vi "FCI_Lip_Gap_Plus_Lip_Level_Pats.vi"(0 "Image":T7(plugin-control), 1 "Calibrated Image":T7, 2 "Ref ROI":T2 {"Contours"."Type" items=["No Selection", "Point", "Line", "Rectangle", "Oval", "Polygon", "Freehand Region", "Annulus", "Unused2", "Unused3", "Broken Line", "Freehand Line", "Rotated Rectangle"]}, 3 "Measurement ROI 1":T2 {"Contours"."Type" items=["No Selection", "Point", "Line", "Rectangle", "Oval", "Polygon", "Freehand Region", "Annulus", "Unused2", "Unused3", "Broken Line", "Freehand Line", "Rotated Rectangle"]}, 4 "Measurement ROI 2":T2 {"Contours"."Type" items=["No Selection", "Point", "Line", "Rectangle", "Oval", "Polygon", "Freehand Region", "Annulus", "Unused2", "Unused3", "Broken Line", "Freehand Line", "Rotated Rectangle"]}, 5 "Line Options Ref ROI":T5={"Number of Lines"=1, "Type"=enum."First Edge Rake", "Min. Score"=10.0, "Max. Score"=1000.0, "Orientation"=0.0, "Angle Range"=45.0, "Angle Tolerance"=1.0, "Step Size"=5, "Min. SNR (db)"=0.0, "Min. Points (%)"=25.0, "Hough Iterations"=5} {"Min. Points (%)" min=0.0 max=100.0; "Min. SNR (db)" min=0.0; "Max. Score" min=0.0 max=1024.0; "Min. Score" min=0.0 max=1024.0 step=1.0}, 6 "Search Direction Ref ROI":u32=2, 7 "error in (no error)":errorcluster, 8 "Search Direction ROI 1":u16(ring) items=["Left To Right", "Right To Left", "Top To Bottom", "Bottom To Top"], 9 "Edge Options ROI 1":T3={"Edge Polarity"=0, "Kernel Size"=3, "Width"=3, "Minimum Edge Strength"=50.0, "Interpolation Type"=enum."Zero Order", "Data Processing Method"=enum."Average"} {"Edge Polarity" items=["All Edges", "Rising Edges", "Falling Edges"]; "Minimum Edge Strength" format="%.2f"; "Width" step=2; "Kernel Size" step=2}, 10 "Search Direction ROI 2":u16(ring)=2 items=["Left To Right", "Right To Left", "Top To Bottom", "Bottom To Top"], 11 "Process ROI 2":T1(ring), 12 "Step Size ROI 2":u32=2, 13 "Edge Options Ref ROI":T3={"Edge Polarity"=0, "Kernel Size"=3, "Width"=3, "Minimum Edge Strength"=40.0, "Interpolation Type"=enum."Zero Order", "Data Processing Method"=enum."Average"} {"Edge Polarity" items=["All Edges", "Rising Edges", "Falling Edges"]; "Minimum Edge Strength" format="%.2f"; "Width" step=2; "Kernel Size" step=2}) -> (20 "Real World Lip Level":sgl, 27 "error IO":errorcluster)   [LabVIEW 2019, in "Algorithm.lvclass"]
uses:
  FrameworkOverrides/Algorithm.lvclass
  <vilib>/vision/NI_Vision_Development_Module.lvlib
  <vilib>/vision/Measure.llb/Edge Polarity.ctl
  <vilib>/vision/Measure.llb/Edge Options.ctl
  <vilib>/vision/Image Controls.llb/IMAQ Image.ctl
  <vilib>/vision/Measure.llb/Straight Edge Process.ctl
  <vilib>/vision/Measure.llb/Straight Edge Options.ctl
panel:
  out "Y1":sgl
  out "Y2":sgl
  out "Pixel Level Difference":sgl
  out "Point 2":cluster{"X":sgl, "Y":sgl}
  out "Point 1":cluster{"X":sgl, "Y":sgl}
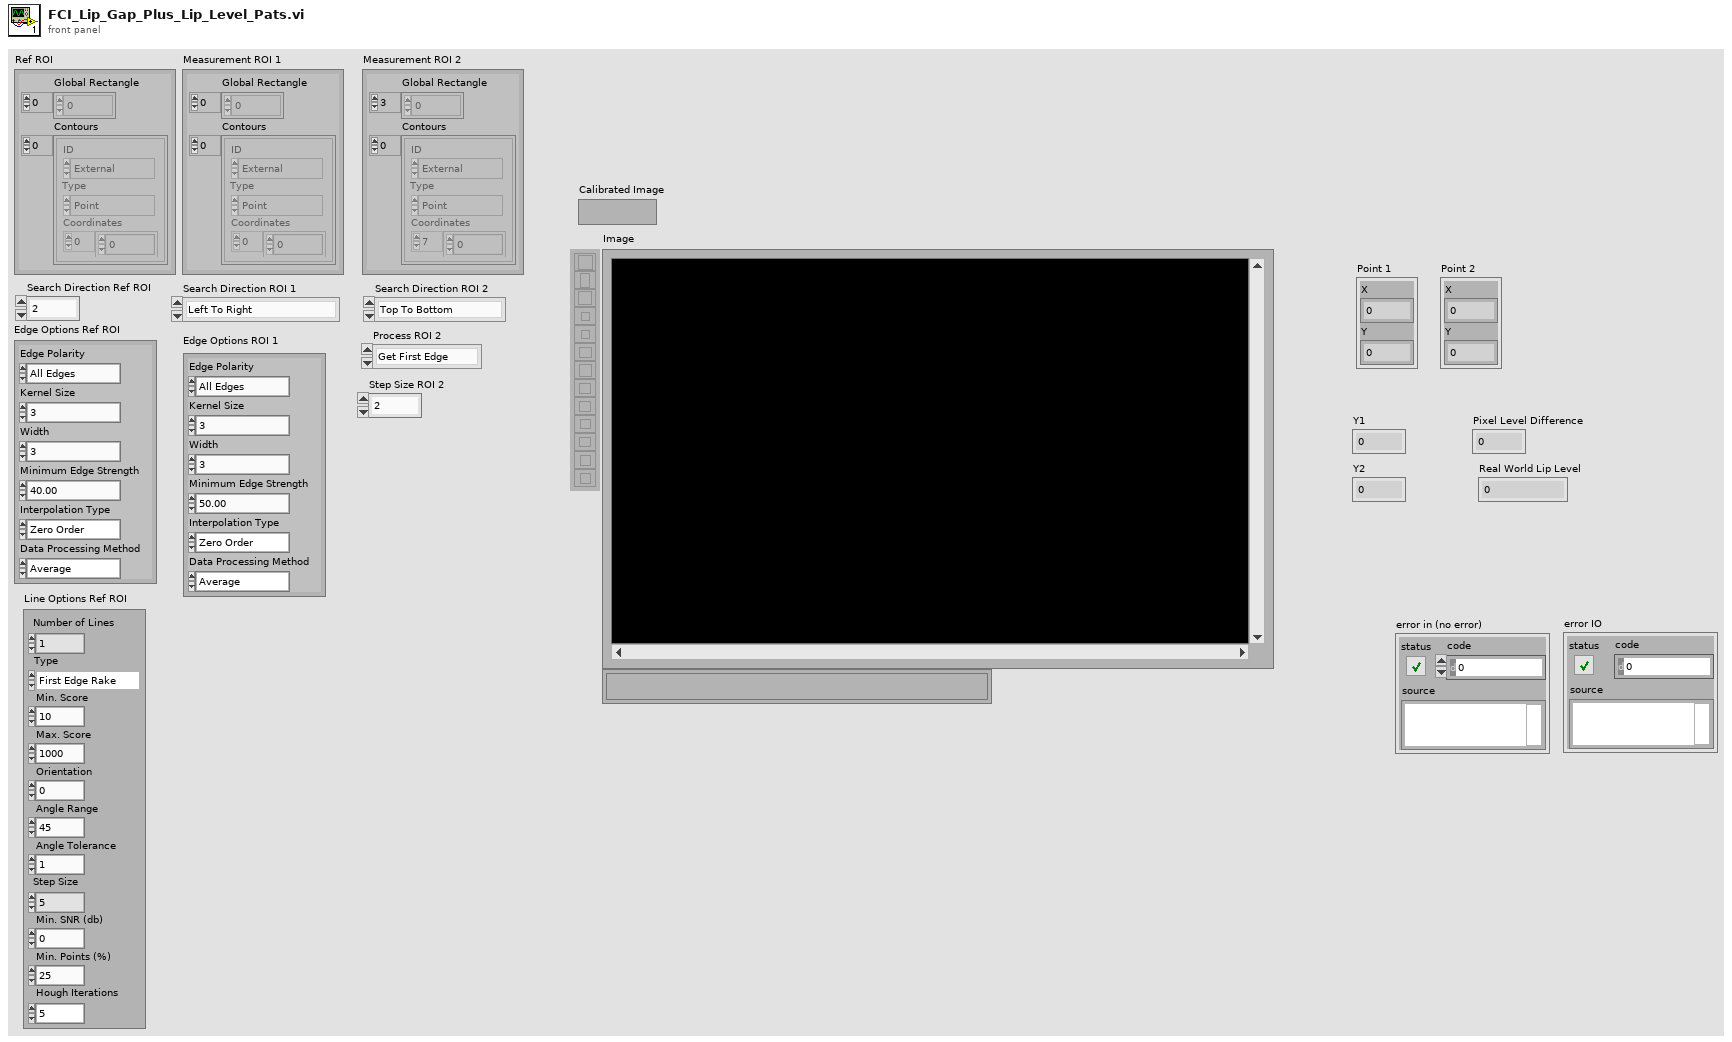
[diagram p1: front panel]
types:
  T1 = enum16{"Get First Edge", "Get First + Last Edge", "Get All Edges", "Get Best Edge"}
  T2 = typedef "ROI Descriptor" = cluster{"Global Rectangle":i32[], "Contours":cluster{"ID":enum32{"External", "Internal"}, "Type":u32, "Coordinates":i32[]}[]}
  T3 = typedef "Edge Options.ctl" = cluster{"Edge Polarity":T4, "Kernel Size":u32, "Width":u32, "Minimum Edge Strength":sgl, "Interpolation Type":enum32{"Zero Order", "Bilinear", "Quadratic", "Cubic", "Bilinear Fixed"}, "Data Processing Method":enum32{"Average", "Median"}}
  T4 = typedef "Edge Polarity.ctl" = u32
  T5 = typedef "Straight Edge Options.ctl" = cluster{"Number of Lines":i32, "Type":T6, "Min. Score":dbl, "Max. Score":dbl, "Orientation":dbl, "Angle Range":dbl, "Angle Tolerance":dbl, "Step Size":u32, "Min. SNR (db)":dbl, "Min. Points (%)":dbl, "Hough Iterations":i32}
  T6 = typedef "Straight Edge Process.ctl" = enum32{"First Edge Rake", "Best Edge Rake", "Hough Edge Rake", "First Edge Projection", "Best Edge Projection"}
  T7 = typedef "IMAQ Image.ctl" = refnum<image>
  T8 = cluster{"Left":dbl, "Top":dbl, "Right":dbl, "Bottom":dbl, "Angle":dbl}
  T9 = cluster{"Search Direction":u32, "Edge Options":T3, "Show Search Area":bool, "Show Search Lines":bool, "Show Edges Found":bool, "Show Result":bool, "Search Area Color":u32, "Search Lines Color":u32, "Edge Locations Color":u32, "Result Color":u32, "Overlay Group Name":string}
  T10 = typedef "IMAQ Rectangle" = cluster{"Left":i32, "Top":i32, "Right":i32, "Bottom":i32, "Rotation":dbl}
  T11 = cluster{"Point1 (Pixels)":cluster{"X":sgl, "Y":sgl}, "Point2 (Pixels)":cluster{"X":sgl, "Y":sgl}, "Point1 (Real-World)":cluster{"X":sgl, "Y":sgl}, "Point2 (Real-World)":cluster{"X":sgl, "Y":sgl}, "Angle (Pixel)":dbl, "Angle (Real-World)":dbl, "Score":dbl, "Straightness":dbl, "Average SNR (db)":dbl, "Calibration Valid":bool}[]
  T12 = cluster{"Point1 (Pixels)":cluster{"X":sgl, "Y":sgl}, "Point2 (Pixels)":cluster{"X":sgl, "Y":sgl}, "Point1 (Real-World)":cluster{"X":sgl, "Y":sgl}, "Point2 (Real-World)":cluster{"X":sgl, "Y":sgl}, "Angle (Pixel)":dbl, "Angle (Real-World)":dbl, "Score":dbl, "Straightness":dbl, "Average SNR (db)":dbl, "Calibration Valid":bool}
  T13 = typedef "Edge New.ctl" = cluster{"Location (Pixel)":cluster{"X":sgl, "Y":sgl}, "Location (Real-World)":cluster{"X":sgl, "Y":sgl}, "Distance (Pixel)":dbl, "Distance (Real-World)":dbl, "Strength":dbl, "Noise":dbl, "Rising?":bool}
  T14 = cluster{cluster{"X":sgl, "Y":sgl}, cluster{"X":sgl, "Y":sgl}}
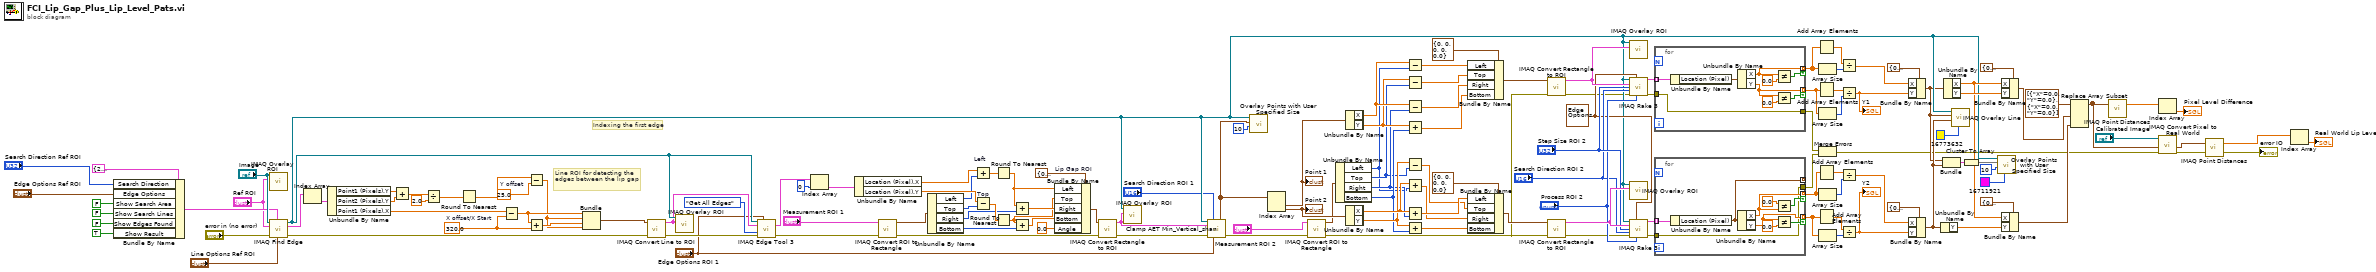
[diagram p0: block diagram]
diagram:
  w56 = sgl 25.0  # Y offset
  w64 = sgl 320.0  # X offset/X Start
  w129 = T3 {"Edge Polarity"=2, "Kernel Size"=3, "Width"=3, "Minimum Edge Strength"=50.0, "Interpolation Type"=enum."Zero Order", "Data Processing Method"=enum."Average"} ("Edge Options")
  # "Indexing the first edge"
  # "Line ROI for detecting the edges between the lip gap"
  n1 = Bundle By Name(cluster=T9 {"Search Direction"=2, "Edge Options"={"Edge Polarity"=0, "Kernel Size"=3, "Width"=3, "Minimum Edge Strength"=40.0, "Interpolation Type"=enum."Zero Order", "Data Processing Method"=enum."Average"}, "Show Search Area"=FALSE, "Show Search Lines"=FALSE, "Show Edges Found"=FALSE, "Show Result"=TRUE, "Search Area Color"=65280, "Search Lines Color"=255, "Edge Locations Color"=16776960, "Result Color"=16711680, "Overlay Group Name"=""} ("Options"), "Search Direction"="Search Direction Ref ROI", "Edge Options"="Edge Options Ref ROI", "Show Search Area"=FALSE, "Show Search Lines"=FALSE, "Show Edges Found"=FALSE, "Show Result"=TRUE) -> (w34:T9)
  n2 = call "IMAQ Overlay ROI"("ROI Descriptor"="Ref ROI", "Image"="Image") -> ()  [unwired: 8 in, 2 out]
  n3 = call "IMAQ Find Edge"("Line Fit Options"="Line Options Ref ROI", "Options"=w34, "error in (no error)"="error in (no error)", "ROI Descriptor"="Ref ROI", "Image"="Image") -> ("error out"=w62:errorcluster, "Straight Edges"=w74:T11, "Image Out"=w80:T7)  [unwired: 3 in, 1 out]
  n4 = Index Array(array=w74) -> (element=w73:T12)  [unwired: 1 in]
  n5 = Unbundle By Name(w73) -> ("Point1 (Pixels).Y"=w72:sgl, "Point2 (Pixels).Y"=w71:sgl, "Point1 (Pixels).X"=w67:sgl)
  n6 = Add(x=w72, y=w71) -> (x+y=w70:sgl)
  n7 = Divide(x=w70, y=sgl 2.0) -> (x/y=w68:sgl)
  n8 = Round To Nearest(number=w68) -> (nearest integer value=w57:sgl)
  n9 = Subtract(x=w67, y=w64) -> (x-y=w66:sgl)
  n10 = Subtract(x=w57, y=w56) -> (x-y=w58:sgl)
  n11 = Add(x=w66, y=w64) -> (x+y=w65:sgl)
  n12 = Bundle(w66, w58, w65, w58) -> (w63:cluster{sgl, sgl, sgl, sgl})  [unwired: 1 in]
  n13 = call "IMAQ Convert Line to ROI"("error in (no error)"=w62, "Line"=w63) -> ("error out"=w61:errorcluster, "ROI Descriptor"=w59:T2)  [unwired: 7 in]
  n14 = call "IMAQ Overlay ROI"("ROI Descriptor"=w59, "Image"=w80) -> ()  [unwired: 8 in, 2 out]
  n15 = call "IMAQ Edge Tool 3"("Image"=w80, "Edge Options"="Edge Options ROI 1", "ROI Descriptor"=w59, "Process"=T1."Get All Edges", "error in (no error)"=w61) -> ("Edge Information"=w55:T13[], "error out"=w21:errorcluster)  [unwired: 6 in, 3 out]
  n16 = Index Array(array=w55, index=0) -> (element=w54:T13)
  n17 = Unbundle By Name(w54) -> ("Location (Pixel).X"=w51:sgl, "Location (Pixel).Y"=w50:sgl)
  n18 = call "IMAQ Convert ROI to Rectangle"("error in (no error)"=w21, "ROI Descriptor"="Measurement ROI 1") -> ("error out"=w20:errorcluster, "Rectangle"=w27:T10)  [unwired: 7 in]
  n19 = Unbundle By Name(w27) -> ("Left"=w26:i32, "Top"=w25:i32, "Right"=w24:i32, "Bottom"=w23:i32)
  n20 = Add "Left"(x=w51, y=w26) -> (x+y=w49:sgl)
  n21 = Subtract "Top"(x=w50, y=w25) -> (x-y=w48:sgl)
  n22 = Round To Nearest(number=w49) -> (nearest integer value=w46:sgl)
  n23 = Round To Nearest(number=w48) -> (nearest integer value=w44:sgl)
  n24 = Add(x=w46, y=w24) -> (x+y=w45:sgl)
  n25 = Add(x=w44, y=w23) -> (x+y=w43:sgl)
  n26 = Bundle By Name "Lip Gap ROI"(cluster=T8 {"Left"=0.0, "Top"=0.0, "Right"=0.0, "Bottom"=0.0, "Angle"=0.0} ("input cluster"), "Left"=w46, "Top"=w44, "Right"=w45, "Bottom"=w43, "Angle"=0.0) -> (w47:T8)
  n27 = call "IMAQ Convert Rectangle to ROI"("error in (no error)"=w20, "Rectangle"=w47) -> ("error out"=w42:errorcluster, "ROI Descriptor"=w41:T2)  [unwired: 7 in]
  n28 = call "IMAQ Overlay ROI"("ROI Descriptor"=w41, "Image"=w80) -> ()  [unwired: 8 in, 2 out]
  n29 = call "Clamp AET Min_Vertical_shan.vi"("Image"=w80, "Scanning axis"="Search Direction ROI 1", "ROI Descriptor"=w41, "error in (no error)"=w42, "Edge Options"="Edge Options ROI 1") -> ("Edge Coordinates"=w141:cluster{"X":sgl, "Y":sgl}[], "error out"=w9:errorcluster)  [unwired: 4 in, 5 out]
  n30 = call "Overlay Points with User Specified Size.vi"("Point Diameter (5)"=u32 10, "Points"=w141, "Image In"=w80) -> ()  [unwired: 7 in, 2 out]
  n31 = Index Array(array=w141) -> (element #1=w140:cluster{"X":sgl, "Y":sgl}, element #2=w137:cluster{"X":sgl, "Y":sgl})  [unwired: 2 in]
  "Point 1" <- w140
  "Point 2" <- w137
  n32 = call "IMAQ Convert ROI to Rectangle"("error in (no error)"=w9, "ROI Descriptor"="Measurement ROI 2") -> ("error out"=w8:errorcluster, "Rectangle"=w7:T10)  [unwired: 7 in]
  n33 = Unbundle By Name(w7) -> ("Left"=w3:i32, "Top"=w4:i32, "Right"=w5:i32, "Bottom"=w6:i32)
  n34 = Unbundle By Name(w140) -> ("X"=w90:sgl, "Y"=w81:sgl)
  n35 = Unbundle By Name(w137) -> ("X"=w86:sgl, "Y"=w84:sgl)
  n36 = Subtract(x=w90, y=w3) -> (x-y=w91:sgl)
  n37 = Subtract(x=w81, y=w4) -> (x-y=w85:sgl)
  n38 = Subtract(x=w90, y=w5) -> (x-y=w89:sgl)
  n39 = Add(x=w81, y=w6) -> (x+y=w82:sgl)
  n40 = Subtract(x=w84, y=w4) -> (x-y=w83:sgl)
  n41 = Add(x=w86, y=w3) -> (x+y=w2:sgl)
  n42 = Add(x=w86, y=w5) -> (x+y=w88:sgl)
  n43 = Add(x=w84, y=w6) -> (x+y=w87:sgl)
  n44 = Bundle By Name(cluster=T10 {"Left"=0, "Top"=0, "Right"=0, "Bottom"=0, "Rotation"=0.0} ("Rectangle"), "Left"=w91, "Top"=w85, "Right"=w89, "Bottom"=w82) -> (w138:T10)
  n45 = Bundle By Name(cluster=T10 {"Left"=0, "Top"=0, "Right"=0, "Bottom"=0, "Rotation"=0.0} ("Rectangle"), "Left"=w88, "Top"=w83, "Right"=w2, "Bottom"=w87) -> (w135:T10)
  n46 = call "IMAQ Convert Rectangle to ROI"("error in (no error)"=w8, "Rectangle"=w138) -> ("error out"=w17:errorcluster, "ROI Descriptor"=w134:T2)  [unwired: 7 in]
  n47 = call "IMAQ Convert Rectangle to ROI"("error in (no error)"=w8, "Rectangle"=w135) -> ("error out"=w16:errorcluster, "ROI Descriptor"=w133:T2)  [unwired: 7 in]
  n48 = call "IMAQ Overlay ROI"("ROI Descriptor"=w134, "Image"=w80) -> ()  [unwired: 8 in, 2 out]
  n49 = call "IMAQ Rake 3"("Image"=w80, "Edge Options"=w129, "ROI Descriptor"=w134, "Step Size"="Step Size ROI 2", "Scan Direction"="Search Direction ROI 2", "error in (no error)"=w17, "Process"="Process ROI 2") -> ("First Edges"=w128:T13[], "error out"=w15:errorcluster)  [unwired: 5 in, 2 out]
  n50 = call "IMAQ Overlay ROI"("ROI Descriptor"=w133, "Image"=w80) -> ()  [unwired: 8 in, 2 out]
  n51 = call "IMAQ Rake 3"("Image"=w80, "Edge Options"=w129, "ROI Descriptor"=w133, "Step Size"="Step Size ROI 2", "Scan Direction"="Search Direction ROI 2", "error in (no error)"=w16, "Process"="Process ROI 2") -> ("First Edges"=w127:T13[], "error out"=w14:errorcluster)  [unwired: 5 in, 2 out]
  n52 = for {
    tunnel: w128 -> [w152] mode=indexing
    tunnel: [w148] -> w117 mode=indexing if=w146
    tunnel: [w147] -> w112 mode=indexing if=w145
    tunnel: w15 -> [w144]
    tunnel: [w144] -> w13
    n53 = Unbundle By Name(w152) -> ("Location (Pixel)"=w150:cluster{"X":sgl, "Y":sgl})
    n54 = Unbundle By Name(w150) -> ("X"=w148:sgl, "Y"=w147:sgl)
    n55 = Not Equal?(x=w148, y=sgl 0.0) -> (x != y?=w146:bool)
    n56 = Not Equal?(x=w147, y=sgl 0.0) -> (x != y?=w145:bool)
  }
  n57 = for {
    tunnel: w127 -> [w161] mode=indexing
    tunnel: [w155] -> w107 mode=indexing if=w159
    tunnel: [w158] -> _ mode=indexing
    tunnel: [w154] -> w106 mode=indexing if=w157
    tunnel: w14 -> [w153]
    tunnel: [w153] -> w12
    n58 = Unbundle By Name(w161) -> ("Location (Pixel)"=w158:cluster{"X":sgl, "Y":sgl})
    n59 = Unbundle By Name(w158) -> ("X"=w155:sgl, "Y"=w154:sgl)
    n60 = Not Equal?(x=sgl 0.0 ("y"), y=w155) -> (x != y?=w159:bool)
    n61 = Not Equal?(x=w154, y=0.0) -> (x != y?=w157:bool)
  }
  n62 = Add Array Elements(numeric array=w117) -> (sum=w116:sgl)
  n63 = Add Array Elements(numeric array=w112) -> (sum=w113:sgl)
  n64 = Add Array Elements(numeric array=w107) -> (sum=w111:sgl)
  n65 = Add Array Elements(numeric array=w106) -> (sum=w108:sgl)
  n66 = Array Size(array=w117) -> (size(s)=w115:i32)
  n67 = Array Size(array=w112) -> (size(s)=w114:i32)
  n68 = Merge Errors(w13, w12) -> (w11:errorcluster)
  n69 = Array Size(array=w107) -> (size(s)=w110:i32)
  n70 = Array Size(array=w106) -> (size(s)=w109:i32)
  n71 = Divide(x=w116, y=w115) -> (x/y=w104:sgl)
  n72 = Divide(x=w113, y=w114) -> (x/y=w100:sgl)
  "Y1" <- w100
  n73 = Divide(x=w111, y=w110) -> (x/y=w102:sgl)
  n74 = Divide(x=w108, y=w109) -> (x/y=w101:sgl)
  "Y2" <- w101
  n75 = Bundle By Name(cluster=cluster{"X":sgl, "Y":sgl} {"X"=0.0, "Y"=0.0}, "X"=w104, "Y"=w100) -> (w78:cluster{"X":sgl, "Y":sgl})
  n76 = Bundle By Name(cluster=cluster{"X":sgl, "Y":sgl} {"X"=0.0, "Y"=0.0}, "X"=w102, "Y"=w101) -> (w79:cluster{"X":sgl, "Y":sgl})
  n77 = Unbundle By Name(w79) -> ("Y"=w95:sgl)
  n78 = Bundle(w78, w79) -> (w94:T14)  [unwired: 1 in]
  n79 = Unbundle By Name(w78) -> ("X"=w96:sgl, "Y"=w97:sgl)
  n80 = call "IMAQ Overlay Line"("Color"=u32 16773632, "End Point"=w79, "Start Point"=w78, "Image"=w80) -> ()  [unwired: 6 in, 2 out]
  n81 = Cluster To Array(cluster=w94) -> (array=w1:cluster{"X":sgl, "Y":sgl}[])
  n82 = call "Overlay Points with User Specified Size.vi"("Color"=u32 16711921, "Point Diameter (5)"=u32 10, "Points"=w1, "Image In"=w80) -> ()  [unwired: 6 in, 2 out]
  n83 = Bundle By Name(cluster=cluster{"X":sgl, "Y":sgl} {"X"=0.0, "Y"=0.0}, "X"=w96, "Y"=w97) -> (w93:cluster{"X":sgl, "Y":sgl})
  n84 = Bundle By Name(cluster=cluster{"X":sgl, "Y":sgl} {"X"=0.0, "Y"=0.0}, "X"=w96, "Y"=w95) -> (w92:cluster{"X":sgl, "Y":sgl})
  n85 = Replace Array Subset(array=cluster{"X":sgl, "Y":sgl}[] [{"X"=0.0, "Y"=0.0}, {"X"=0.0, "Y"=0.0}] ("Points"), new element #1=w93, new element #2=w92) -> (w121:cluster{"X":sgl, "Y":sgl}[])  [unwired: 2 in]
  n86 = call "IMAQ Point Distances"("Points"=w121) -> ("Distances"=w125:sgl[])  [unwired: 4 in, 1 out]
  n87 = Index Array(array=w125) -> (element=→"Pixel Level Difference":sgl)  [unwired: 1 in]
  n88 = call "IMAQ Convert Pixel to Real World"("error in (no error)"=w11, "Array of Pixel Coordinates"=w121, "Calibrated Image"="Calibrated Image") -> ("error out"=w18:errorcluster, "Array of Real World Coordinates"=w118:cluster{"X":sgl, "Y":sgl}[])  [unwired: 3 in, 4 out]
  n89 = call "IMAQ Point Distances"("Points"=w118, "error in (no error)"=w18) -> ("Distances"=w119:sgl[], "error out"=→"error IO":errorcluster)  [unwired: 3 in]
  n90 = Index Array(array=w119) -> (element=→"Real World Lip Level":sgl)  [unwired: 1 in]
